vi "N5765A_WaitforPowerDown.vi"(5 "Timeout (s)":dbl, 7 "Current Threshold (A)":dbl, 8 "error in (no error)":errorcluster, 11 "VISA resource name":refnum<visa-resource-name>="PS2") -> (0 "error out":errorcluster)   [LabVIEW 2015]
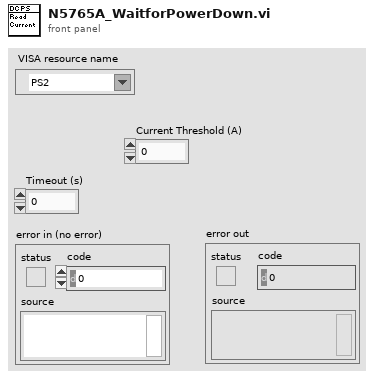
[diagram p1: front panel]
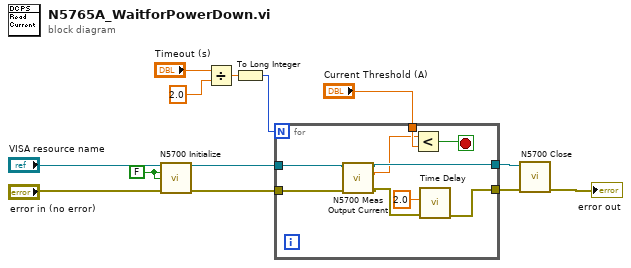
[diagram p0: block diagram]
diagram:
  w4 = FALSE ("ID Query? (T: Yes)")
  n1 = call <instrlib>:"N5700 Initialize.vi"("VISA name"="VISA resource name", "ID Query (T)"=w4, "Reset (T)"=w4, "error in (no error)"="error in (no error)") -> ("VISA out"=w7:refnum<visa-resource-name>, "error out"=w6:errorcluster)  [unwired: 10 in]
  n2 = Divide(x="Timeout (s)", y=2.0) -> (x/y=w10:dbl)
  n3 = To Long Integer(number=w10) -> (32bit integer=w9:i32)
  n4 = for {
    N: w9 -> [_]
    tunnel: w7 -> [w16]
    tunnel: w6 -> [w18]
    tunnel: [w21] -> w2
    tunnel: [w15] -> w3
    tunnel: "Current Threshold (A)" -> [w20]
    stop <- w19 stop-if-true
    n5 = call <instrlib>:"N5700 Meas Output Current.vi"("error"=w18, "VISA"=w16) -> ("error out"=w17:errorcluster, "Output Current"=w14:dbl, "VISA out"=w15:refnum<visa-resource-name>)  [unwired: 4 in]
    n6 = Less?(x=w14, y=w20) -> (x < y?=w19:bool)
    n7 = call "Time Delay"("error in (no error)"=w17, "Delay Time (s)"=2.0) -> ("error out"=w21:errorcluster)  [unwired: 9 in]
  }
  n8 = call <instrlib>:"N5700 Close.vi"("error"=w2, "VISA name"=w3) -> ("error out"=→"error out":errorcluster)  [unwired: 6 in]
